vi "Constants.vi"() -> ()   [LabVIEW 2019, in "UDP-Custom-Device Shared.lvlib"]
doc: "Use this Global VI to access the GUIDs assigned to the page resources of the Custom Device."
uses:
  UDP-Custom-Device Shared.lvlib
panel:
  in  "Tab Control":T1(tab)=enum."Main Page"
  in  "GUID - Tx Channel Page":string="4fe98813-0d2f-43b7-911c-1a5a6e2d5286"
  in  "GUID - Tx Channel Section":string="110650c2-dfee-41b8-9f4d-56262735f1a2"
  in  "GUID - Buffered Receive Packet":string="0b9a6620-1662-48a0-94bf-5c5feb9252a9"
  in  "GUID - Buffered Transmit Packet":string="82671a20-3042-4259-849c-bf21b4eca2c0"
  in  "GUID - Tx Timestamp Channel Page":string="110650c2-dfee-41b8-9f4d-56262735f1a2"
  in  "GUID - Tx Channel Config Page":string="7134e672-8954-4c1e-90f9-b2ce44aa937f"
  in  "GUID - Rx Channel Section":string="b8f54c24-25be-4871-8286-2c037e7fae7b"
  in  "GUID - Rx Channel Config Page":string="d07b28d3-a93a-42af-82ec-413131de3387"
  in  "GUID - Tx Packet Page":string="af86c4de-d36a-4f1e-b637-4db21d1b2000"
  in  "GUID - Rx Packet Page":string="fe00aa1c-0d2c-4749-801e-e5de1d827245"
  in  "GUID - Diagnostics Channel Page":string="dbe1565a-647c-4128-a5fd-e9726cfe8b31"
  in  "GUID - Diagnostics Section Page":string="4fe98813-0d2f-43b7-911c-1a5a6e2d5286"
  in  "GUID - Rx Channel Page":string="8ede79f1-e06f-41dd-88ab-5074f11d4bb7"
  in  "GUID - Tx Section Page":string="83990986-7c5f-4a4f-9521-e5ef95a941a7"
  in  "GUID - Rx Section Page":string="e4cf9946-87d0-45cb-83bc-815ce28b6d77"
  in  "GUID - UDP-Custom-Device":string="1dbe19ca-57a1-40f3-b205-33efa5cbd18f"
  in  "GUID - Remove Packet RTM":string="d100fb3b-4693-4e75-a071-1f9383acb0bd"
  in  "GUID - Add Packet RTM":string="92cecc98-59fe-421e-b292-1ac1a1e86434"
  in  "GUID - Import Config RTM":string="a9527afc-c1bc-42ef-a605-ac6813829a8e"
  in  "GUID - Export Config RTM":string="8a091f2f-f6f5-4838-b57c-7ff242367d6e"
  in  "GUID - Apply Tx Config RTM":string="4e2a141b-9661-4348-be05-fbd002a512fc"
  in  "GUID - Apply Rx Config RTM":string="c6628006-2c41-4618-9061-c84e9f8f3bb9"
  in  "GUID - Add Rx Channel RTM":string="05d99361-a9e2-444c-9f7f-46d513041ad0"
  in  "GUID - Remove Rx Channel RTM":string="dec96e15-7a09-4d9c-9a7c-4429dad53fd3"
  in  "Main - Export File Location":string="Main.ExportFileLocation"
  in  "Main - Export to File Status":string="Main.ExportToFileStatus"
  in  "Main - TimeStamp Ref":string="Main.TimeStampRef"
  in  "Compiled.Settings":string="Compiled.Settings"
  in  "Section - Packet Names":string="Section.PacketNames"
  in  "Section - Selected Packets":string="Section.SelectedPackets"
  in  "Section - Packet Refs":string="Section.PacketRefs"
  in  "Section - Packet IDs":string="Section.PacketIDs"
  in  "Packet - Thread Management":string="Packet.ThreadManagement"
  in  "Packet - Priority":string="Packet.Priority"
  in  "Packet - Target Processor":string="Packet.TargetProcessor"
  in  "Packet - Debug Mode":string="Packet.DebugMode"
  in  "Packet - Multicast IP":string="Packet.MulticastIP"
  in  "Packet - Multicast":string="Packet.Multicast"
  in  "Packet - Selected Channels":string="Packet.SelectedChannels"
  in  "Packet - Local Port":string="Packet.LocalPort"
  in  "Packet - Endianness":string="Packet.Endianness"
  in  "Packet - Packet ID":string="Packet.PacketID"
  in  "Packet - Local NIC IP":string="Packet.LocalNICIP"
  in  "Packet - Header Info":string="Packet.HeaderInfo"
  in  "Packet - Channel Refs":string="Packet.ChannelRefs"
  in  "Packet - Channel Paths":string="Packet.ChannelPaths"
  in  "Packet - Channel Names":string="Packet.ChannelNames"
  in  "Packet - Auto-Assign NIC":string="Packet.AutoAssignNIC"
  in  "Rx Packet - New Data Option":string="RxPacket.NewDataOption"
  in  "Rx Packet - Channel Dest Path":string="RxPacket.ChannelDestination Path"
  in  "Rx Packet - Read Timeout":string="RxPacket.ReadTimeout"
  in  "Rx Packet - Diagnostics En?":string="DiagnosticsEnabled"
  in  "Tx Packet - Loop Period":string="TxPacket.LoopPeriod"
  in  "Tx Packet - Thread Sync":string="TxPacket.ThreadSync"
  in  "Tx Packet - Transmit Echo Option":string="TxPacket.TransmitEchoOption"
  in  "Tx Packet - Transmit Option":string="TxPacket.TransmitOption"
  in  "Tx Packet - Port as Channel":string="TxPacket.PortAsChannel"
  in  "Tx Packet - TTL":string="TxPacket.TTL"
  in  "Tx Packet - Always Transmit":string="TxPacket.AlwaysTransmit"
  in  "Tx Packet - Timestamp Ref":string="TxPacket.TimestampRef"
  in  "Tx Packet - Data Types":string="TxPacket.DataTypes"
  in  "Del - Tx Remove Channel Button ID":string="NIVS_UDPDataLink_Tx_RemoveChannels"
  in  "Tx Packet - Destination IP":string="TxPacket.DestinationIP"
  in  "Tx Packet - Decimation":string="TxPacket.Decimation"
  in  "Tx Packet - Destination Port":string="TxPacket.DestinationPort"
  in  "Tx Packet - Diagnostics En?":string="DiagnosticsEnabled"
  in  "Rx Channel Section - Dependent Nodes":string="RxChannels.DependentNodes"
  in  "Tx Channel Section - Dependent Nodes":string="TxChannels.DependentNodes"
  in  "Rx Channel - Destination Ref":string="RxPacket.ChannelDestinationRef"
  in  "Rx Channel - Data Type":string="RxPacket.ChannelDestinationRef"
  in  "Tx Channel - Destination Ref":string="TxPacket.ChannelDestinationRef"
  in  "Tx Channel - Data Type":string="TxPacket.ChannelDestinationRef"
  in  "Channel CFG - Number of Instances":string="ChannelConfig.NumbInstances"
  in  "Channel CFG - Append Channels":string="ChannelConfig.AppendChannels"
  in  "Channel CFG - Selected Channels":string="ChannelConfig.SelChans"
  in  "Channel CFG - Config File":string="ChannelConfig.ConfigPath"
  in  "Buffered Data - Tx Sim Option":string="BufferData.TxSimOption"
  in  "Buffered Data - Tx Buffer Option":string="BufferData.TxBufferOption"
  in  "Buffered Data - Pointer Encoding":string="BufferedData.PointerEncoding"
  in  "Buffered Data - External Buffer":string="BufferedData.ExtBuffer"
  in  "Buffered Data - Prepend Header":string="BufferedData.PrependHeader"
  in  "Buffered Data - Buffer Size":string="BufferedData.BufferSize"
  in  "Buffered Data - Rx Buffer Option":string="BufferData.RxBufferOption"
  # "Main Page Properties"
  # "Shared Section Properties"
  # "Shared Packet Properties"
  # "Rx Packet Properties"
  # "Tx Packet Properties"
  # "Rx Channel Properties"
  # "Tx Channel Properties"
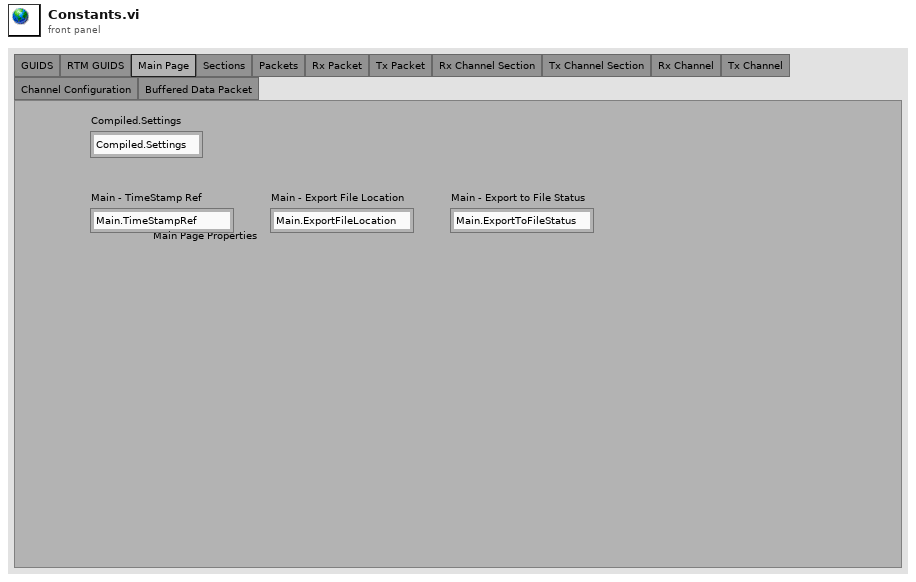
[diagram p1: front panel]
types:
  T1 = enum32{"GUIDS", "RTM GUIDS", "Main Page", "Sections", "Packets", "Rx Packet", "Tx Packet", "Rx Channel Section", "Tx Channel Section", "Rx Channel", "Tx Channel", "Channel Configuration", "Buffered Data Packet"}
diagram:
